vi "GravityCompensation.vi"(1 "Position [deg]":dbl) -> (0 "Current":dbl)   [LabVIEW 2019]
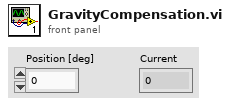
[diagram p1: front panel]
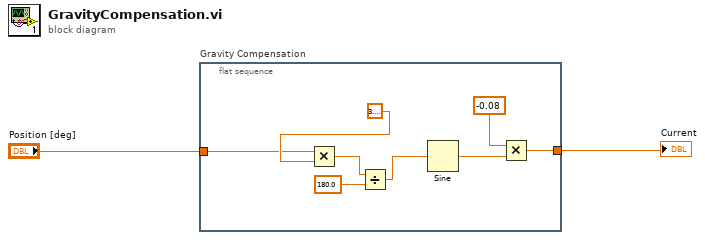
[diagram p0: block diagram]
diagram:
  n1 = flat-sequence "Gravity Compensation" {
    tunnel: [w4] -> w1
    tunnel: "Position [deg]" -> [w3]
    frame #0 {
      n2 = Multiply(x=w3, y=3.141592653589793) -> (x*y=w9:dbl)
      n3 = Divide(x=w9, y=180.0) -> (x/y=w7:dbl)
      n4 = Sine(x=w7) -> (sin(x)=w6:dbl)
      n5 = Multiply(x=-0.08, y=w6) -> (x*y=w4:dbl)
    }
  }
  "Current" <- w1
